vi "Test RS.vi"() -> ()   [LabVIEW 2014]
panel:
  in  "T=growth\nF=back and forth":bool
  out "Numeric":dbl
  out "Axis":i32
  in  "T=extend\nF=contract":bool=TRUE
  in  "# of Step":dbl=10.0
  in  "Dwell time (ms)":dbl=200.0
  in  "Step (nm)":dbl=10.0
  in  "T=X\nF=Y":bool=TRUE
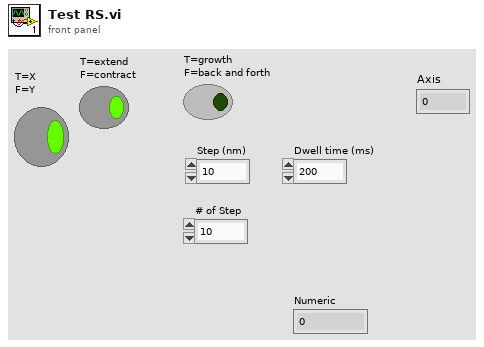
[diagram p1: front panel]
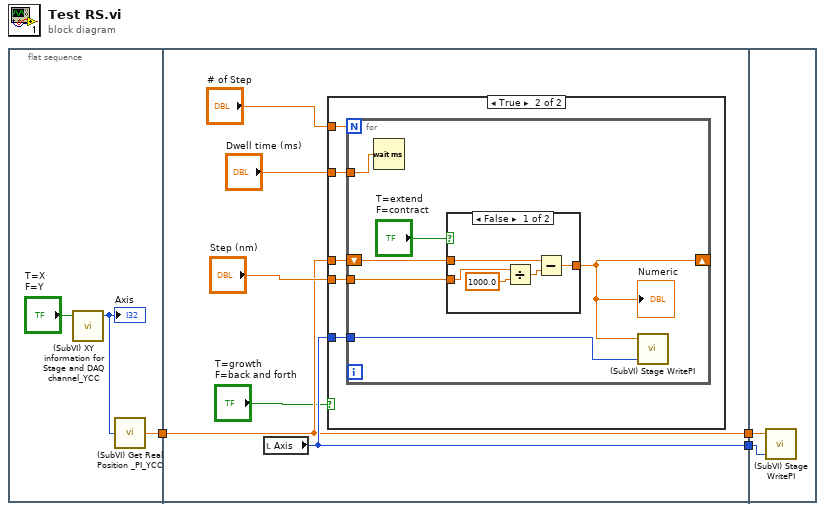
[diagram p0: block diagram]
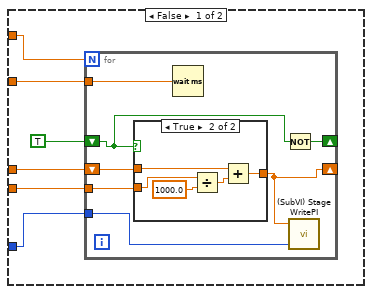
[diagram p2: hidden frame]
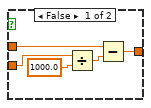
[diagram p3: hidden frame]
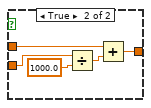
[diagram p4: hidden frame]
diagram:
  n1 = flat-sequence {
    tunnel: [w4] -> w3
    tunnel: w3 -> [w8]
    tunnel: [w9] -> w2
    tunnel: [w8] -> w1
    tunnel: w2 -> [w58]
    tunnel: w1 -> [w57]
    frame #0 {
      n2 = call "(SubVI) XY information for Stage and DAQ channel_YCC.vi"("T=X\nF=Y"="T=X\nF=Y") -> ("Axis"=w5:i32)  [unwired: 3 in, 1 out]
      "Axis" <- w5
      n3 = call "(SubVI) Get Real Position _PI_YCC.vi"("Axis"=w5) -> ("Real Current Commanded position (um)"=w4:dbl)  [unwired: 4 in]
    }
    frame #1 {
      n4 = local read "Axis"() -> (w9:i32)
      n5 = case shown="True" "T=growth\nF=back and forth" {
        tunnel: "# of Step" -> [w14 w40]
        tunnel: "Step (nm)" -> [w17 w39]
        tunnel: "Dwell time (ms)" -> [w13 w38]
        tunnel: w9 -> [w15 w37]
        tunnel: w8 -> [w18 w36]
        frame False {
          n6 = for {
            N: w14 -> [_]
            tunnel: w17 -> [w24]
            shift-right: [w23] -> _
            shift-left: TRUE -> [w22]
            tunnel: w15 -> [w21]
            tunnel: w13 -> [w20]
            shift-right: [w19] -> _
            shift-left: w18 -> [w25]
            n7 = case shown="True" w22 {
              tunnel: w25 -> [w30 w34]
              tunnel: w24 -> [w29 w33]
              tunnel: [w26 w31] -> w19
              frame False {
                n8 = Divide(x=w29, y=1000.0) -> (x/y=w27:dbl)
                n9 = Subtract(x=w30, y=w27) -> (x-y=w26:dbl)
              }
              frame True {
                n10 = Divide(x=w33, y=1000.0) -> (x/y=w32:dbl)
                n11 = Add(x=w34, y=w32) -> (x+y=w31:dbl)
              }
            }
            n12 = Wait (ms)(milliseconds to wait=w20) -> ()  [unwired: 1 out]
            n13 = Not(x=w22) -> (.not. x?=w23:bool)
            n14 = call "(SubVI) Stage WritePI.vi"("axis"=w21, "position"=w19) -> ()  [unwired: 4 in]
          }
        }
        frame True {
          n15 = for {
            N: w40 -> [_]
            tunnel: w39 -> [w44]
            tunnel: w37 -> [w43]
            tunnel: w38 -> [w42]
            shift-right: [w41] -> _
            shift-left: w36 -> [w45]
            n16 = Wait (ms)(milliseconds to wait=w42) -> ()  [unwired: 1 out]
            n17 = case shown="False" "T=extend\nF=contract" {
              tunnel: w45 -> [w51 w55]
              tunnel: w44 -> [w50 w54]
              tunnel: [w47 w52] -> w41
              frame False {
                n18 = Divide(x=w50, y=1000.0) -> (x/y=w48:dbl)
                n19 = Subtract(x=w51, y=w48) -> (x-y=w47:dbl)
              }
              frame True {
                n20 = Divide(x=w54, y=1000.0) -> (x/y=w53:dbl)
                n21 = Add(x=w55, y=w53) -> (x+y=w52:dbl)
              }
            }
            "Numeric" <- w41
            n22 = call "(SubVI) Stage WritePI.vi"("axis"=w43, "position"=w41) -> ()  [unwired: 4 in]
          }
        }
      }
    }
    frame #2 {
      n23 = call "(SubVI) Stage WritePI.vi"("axis"=w58, "position"=w57) -> ()  [unwired: 4 in]
    }
  }
